vi "sub_Buffer_main.vi"(8 "error in (no error)":errorcluster caption="错误输入（无错误）", 9 "operation":enum16{"Init", "Update", "Get"}(ring), 10 "index":i32[](array[numeric]), 11 "Buffer in":dbl[](array[numeric])) -> (0 "error out":errorcluster caption="错误输出", 3 "Buffer out":dbl[](array[numeric]))   [LabVIEW 2011]
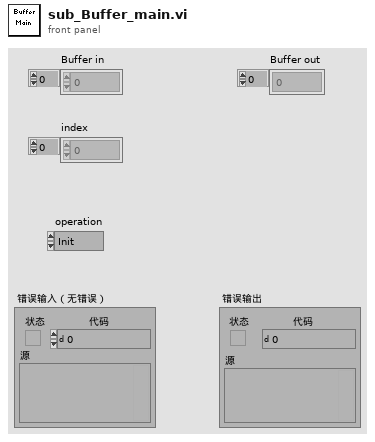
[diagram p1: front panel]
types:
  T1 = cluster{"SPN":u32, "Name":string, "SlotType":enum16{"Unknown Type", "Acceleration", "Angle", "ASCII", "Bool", "Brake Applications", "Bit Field", "Number of bytes", "Capacity, Battery", "Control byte", "Calendar, days", "Calendar, months", "Conductivity", "Count", "Calendar, weeks", "Calendar, years", "Dielectricity", "Direction", "Distance", "Electrical Current", "Economy, gaseous", "Economy, liquid", "Energy", "Electrical Voltage", "Flow rate, gaseous", "Flow rate, liquid", "FMI", "Frequency", "Force", "Fuel Used,gaseous", "Fuel Used, liquid", "Flow rate,volumetric", "Group Function", "Governor gain", "Gear Ratio", "Gear Value", "Identifier", "Inertia", "Intensity, optical", "Kinematic viscosity", "level", "Mass,cargo", "Name (short)", "Name (long)", "OC", "Power, Apparent", "Percent", "Percent,concentration", "Proprietary Data", "position", "Power Factor", "Parts Per Million", "Pressure", "Pressure Rate Change", "Power, Reactive", "Power, Real", "Ratio", "Road Curvature", "Record", "Revolutions", "Source Address", "Specific Gravity", "SPN", "Specific Resistance", "Step", "Transfer Data", "Time", "Temperature", "Torque", "Velocity,angular", "VariantData", "Velocity, linear", "Velocity, magnitude", "Volume", "Velocity, rotational"}, "Unit":enum16{"UnDefined", "%", "1", "1/km", "A", "ASCII", "bin", "bit", "℃", "D", "deg", "deg/s", "g", "Hz", "ID", "kg", "kg/h", "kg/m^2", "km", "km/kg", "km/L", "kPa", "kph", "kW", "kWh", "L", "L/h", "m", "m/h", "m/s", "m/s^2", "m^3/h", "mAh", "min", "mm", "mm^2/s", "Mon", "ms", "mSi/mm", "mW/cm^2", "N", "Nm", "Pa/s", "ppm", "r", "rad/s", "Rat", "Rec", "rpm", "s", "SA", "step", "TF", "V", "VA", "VAr", "W", "Y", "Ωm"}, "Value":variant, "Scaling":dbl, "LowLmt":dbl, "HighLmt":dbl, "Offset":dbl, "Length":u8, "PGN":u32, "Comment":string, "LastUpdate":timestamp}[]
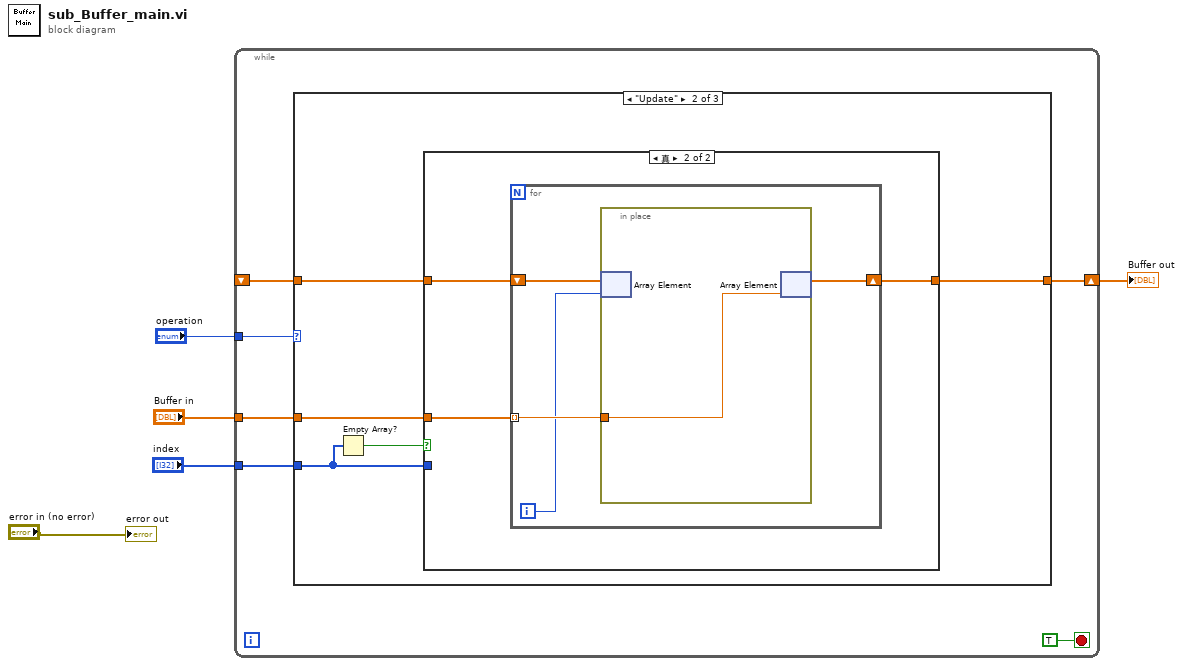
[diagram p0: block diagram]
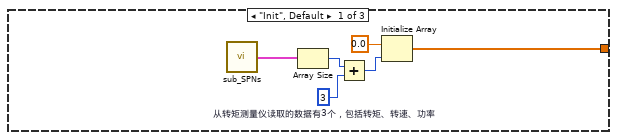
[diagram p2: hidden frame]
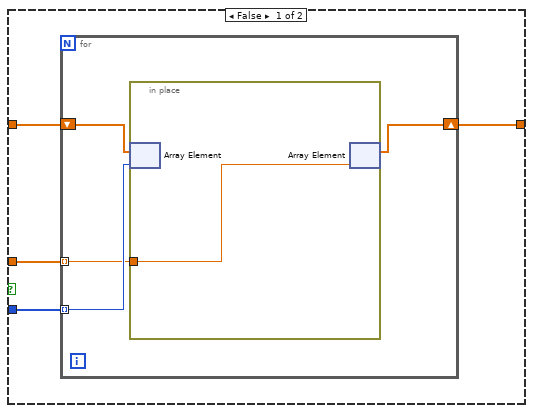
[diagram p3: hidden frame]
diagram:
  n1 = while {
    tunnel: "operation" -> [w10]
    tunnel: "Buffer in" -> [w7]
    shift-right: [w9] -> w1
    shift-left: _ -> [w8]
    tunnel: "index" -> [w6]
    stop <- TRUE stop-if-true
    n2 = case shown="\"Update\"" w10 {
      tunnel: [w13 w20 w40] -> w9
      tunnel: w8 -> [_ w21 w40]
      tunnel: w7 -> [_ w22 _]
      tunnel: w6 -> [_ w19 _]
      frame "Init", Default {
        w16 = 3  # 从转矩测量仪读取的数据有3个，包括转矩、转速、功率
        n3 = call "sub_SPNs.vi"() -> ("SPNs"=w12:T1)
        n4 = Array Size(array=w12) -> (size(s)=w15:i32)
        n5 = Add(x=w15, y=w16) -> (x+y=w14:i32)
        n6 = Initialize Array(0.0, w14) -> (w13:dbl[])
      }
      frame "Update" {
        n7 = Empty Array?(array=w19) -> (empty?=w18:bool)
        n8 = case shown="真" w18 {
          tunnel: w22 -> [w26 w32]
          tunnel: w21 -> [w25 w34]
          tunnel: [w24 w33] -> w20
          tunnel: w19 -> [w23 _]
          frame False {
            n9 = for {
              tunnel: w26 -> [w28] mode=indexing
              tunnel: w23 -> [w29] mode=indexing
              shift-right: [w27] -> w24
              shift-left: w25 -> [w30]
              n10 = in-place {
                in-place-border: w28 -> [w31]
                n11 = in-place-array #1(w30, w29) -> ()  [unwired: 1 out]
                n12 = in-place-array #1(w31) -> (w27:dbl[])  [unwired: 1 out]
              }
            }
          }
          frame True {
            n13 = for {
              shift-right: [w36] -> w33
              shift-left: w34 -> [w38]
              tunnel: w32 -> [w37] mode=indexing
              i -> [w35]
              n14 = in-place {
                in-place-border: w37 -> [w39]
                n15 = in-place-array #2(w38, w35) -> ()  [unwired: 1 out]
                n16 = in-place-array #2(w39) -> (w36:dbl[])  [unwired: 1 out]
              }
            }
          }
        }
      }
      frame "Get" {
      }
    }
  }
  "Buffer out" <- w1
  "error out" <- "error in (no error)"
